vi "test Mutate Device Driver.vi"(8 "error in (no error)":errorcluster, 11 "TestCase in":refnum<class "Embedded Data Logger Unit Tests.lvclass">) -> (0 "error out":errorcluster, 3 "TestCase out":refnum<class "Embedded Data Logger Unit Tests.lvclass">)   [LabVIEW 2027, in "Embedded Data Logger Unit Tests.lvclass"]
uses:
  Embedded Data Logger Unit Tests.lvclass
  C:/Program Files/National Instruments/LabVIEW 2027/vi.lib/addons/_JKI Toolkits/VI Tester/TestCase.llb/TestCase.lvclass
  <vilib>/addons/_JKI Toolkits/VI Tester/TestCase.llb/TestCase.lvclass
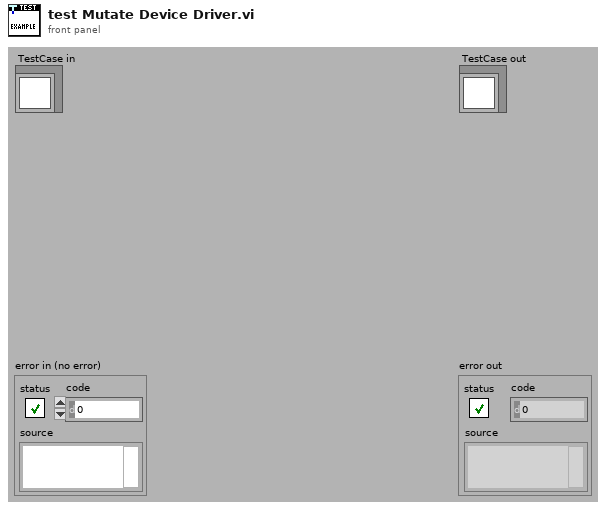
[diagram p1: front panel]
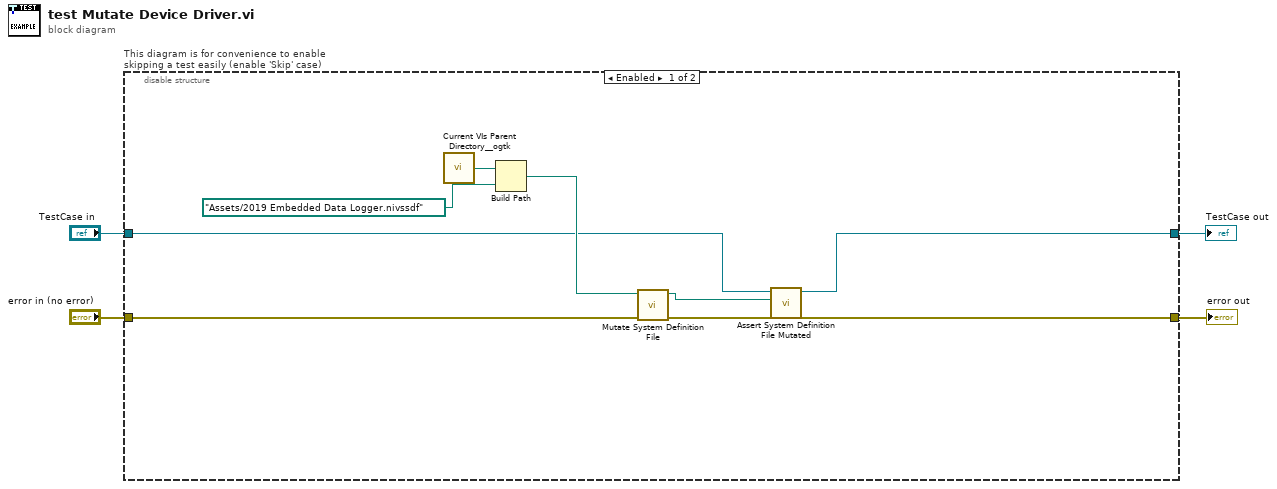
[diagram p0: block diagram]
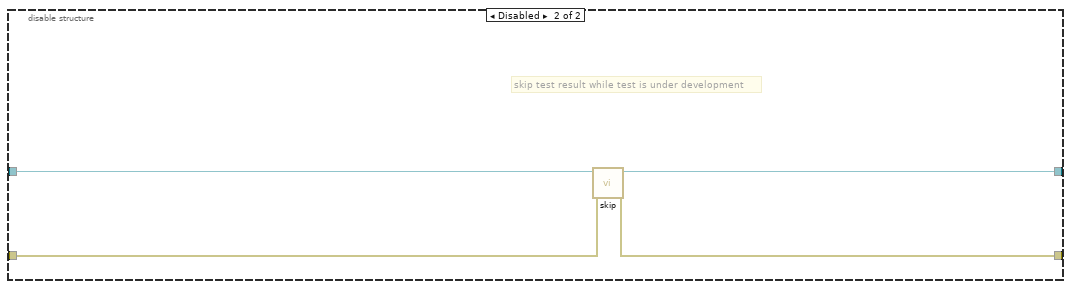
[diagram p2: hidden frame]
diagram:
  n1 = disable-structure "This diagram is for convenience to enable skipping a test easily (enable 'Skip' case)" shown="Enabled" {
    disable-tunnel: "TestCase in" -> [w7 w17]
    disable-tunnel: [w6 w15] -> w1
    disable-tunnel: [w8 w16] -> w3
    disable-tunnel: "error in (no error)" -> [w13 w14]
    frame Enabled {
      n2 = call <userlib>:"Current VIs Parent Directory__ogtk.vi"() -> ("Parent Directory (+ Relative)"=w12:path)  [unwired: 5 in]
      n3 = Build Path(base path=w12, name or relative path=path "Assets/2019 Embedded Data Logger.nivssdf" ("Parent Directory (+ Relative)")) -> (appended path=w11:path)
      n4 = call "Mutate System Definition File.vi"("error in (no error)"=w13, "Original System Definition File"=w11) -> ("error out"=w9:errorcluster, "Mutated System Definition File"=w10:path)  [unwired: 8 in]
      n5 = call "Assert System Definition File Mutated.vi"("error in (no error)"=w9, "Mutated System Definition File"=w10, "Embedded Data Logger Unit Tests in"=w7) -> ("error out"=w8:errorcluster, "Embedded Data Logger Unit Tests out"=w6:refnum<class "Embedded Data Logger Unit Tests.lvclass">)  [unwired: 7 in]
    }
    frame Disabled {
      # "skip test result while test is under development"
      n6 = call <vilib>:"skip.vi"("error in (no error)"=w14, "TestCase in"=w17) -> ("error out"=w16:errorcluster, "TestCase out"=w15:refnum<class "Embedded Data Logger Unit Tests.lvclass">)  [unwired: 8 in]
    }
  }
  "error out" <- w3
  "TestCase out" <- w1
